vi "Event Set Event.vi"(8 "error in (no error)":errorcluster, 10 "Event name":string, 11 "Event DVR in":refnum<data-value>) -> (0 "error out":errorcluster, 3 "Event DVR out":refnum<data-value>)   [LabVIEW 2015, in "MDSplus.lvlib"]
doc: "Issues a new event."
uses:
  MDSplus.lvlib
  Classes/Event_Class/Event.lvclass
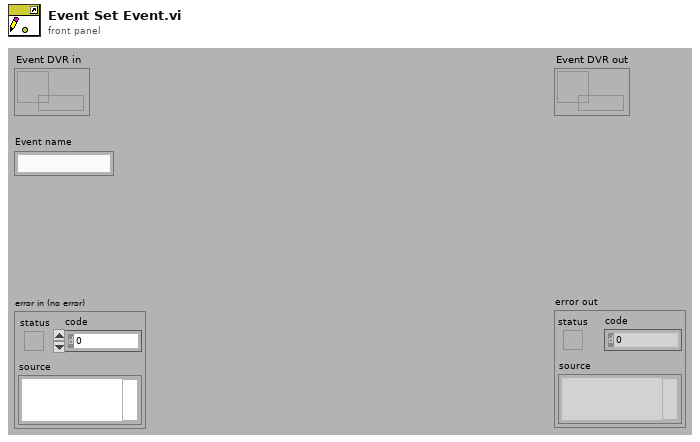
[diagram p1: front panel]
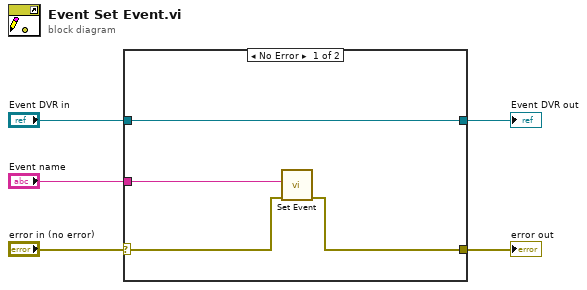
[diagram p0: block diagram]
diagram:
  n1 = case shown="No Error" "error in (no error)" {
    selector: "error in (no error)" -> [w8 w10]
    tunnel: "Event DVR in" -> [w6 w11]
    tunnel: [w7 w10] -> w5
    tunnel: [w6 w11] -> w2
    tunnel: "Event name" -> [w9 _]
    frame No Error {
      n2 = call "Set Event.vi"("error in (no error)"=w8, "Event name"=w9) -> ("error out"=w7:errorcluster)  [unwired: 8 in, 1 out]
    }
    frame Error {
    }
  }
  "error out" <- w5
  "Event DVR out" <- w2
